vi "0x03ReadHoldingRegisters.vi"(6 "Length 2":u16, 8 "error in (no error)":errorcluster, 9 "Register":u16, 10 "Addressc":u8, 11 "Modbus in":refnum<class "Modbus.lvclass">) -> (0 "error out":errorcluster, 2 "Frame":string, 3 "Modbus out":refnum<class "Modbus.lvclass">)   [LabVIEW 2015, in "ModBUS.lvlib" / "Modbus.lvclass"]
uses:
  Modbus.lvclass
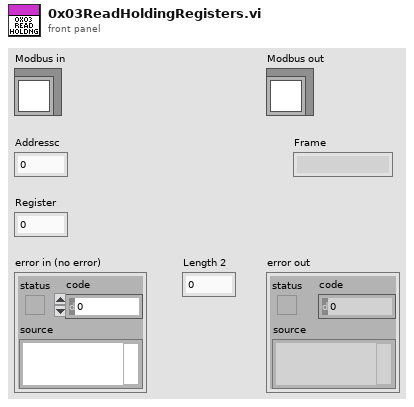
[diagram p1: front panel]
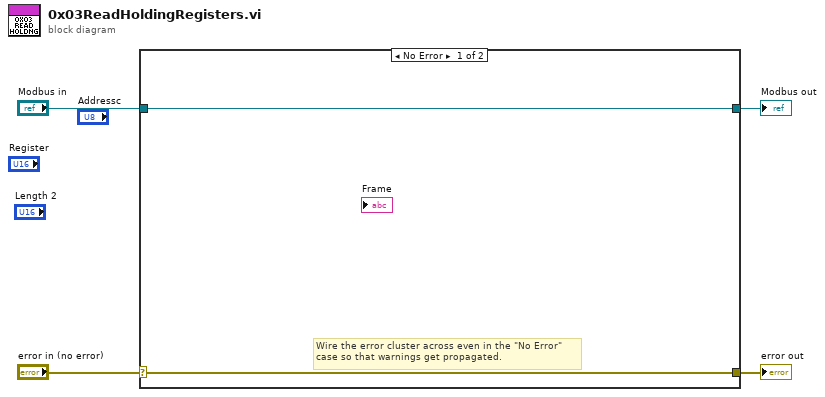
[diagram p0: block diagram]
diagram:
  n1 = case shown="No Error" "error in (no error)" {
    selector: "error in (no error)" -> [w5 w8]
    tunnel: [w5 w8] -> w3
    tunnel: [w6 w7] -> w1
    tunnel: "Modbus in" -> [w6 w7]
    frame No Error {
      # "Wire the error cluster across even in the \"No Error\"\ncase so that warnings get propagated."
    }
    frame Error {
    }
  }
  "error out" <- w3
  "Modbus out" <- w1
